vi "Register for Event.vi"(4 "Error In":errorcluster) -> (0 "Error Out":errorcluster, 3 "sys":refnum<event-registration>)   [LabVIEW 2015, in "ude_Handle Errors.lvlib"]
uses:
  ude_Handle Errors.lvlib
  Event Data.ctl
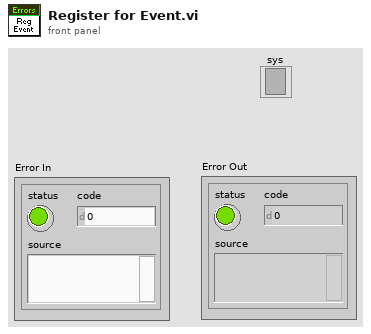
[diagram p1: front panel]
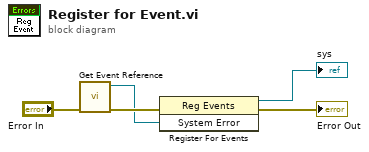
[diagram p0: block diagram]
diagram:
  n1 = call "Get Event Reference.vi"("error in (no error)"="Error In") -> ("error out"=w4:errorcluster, "System Error"=w3:refnum<user-event>)  [unwired: 5 in]
  n2 = register-events(error in=w4, w3) -> (reference out=→"sys":refnum<event-registration>, error out=→"Error Out":errorcluster)  [unwired: 1 in]
